vi "Limit Error.vi"(1 "Array":u8[](array[numeric])) -> (0 "LIMIT ERROR":bool)   [LabVIEW 2015]
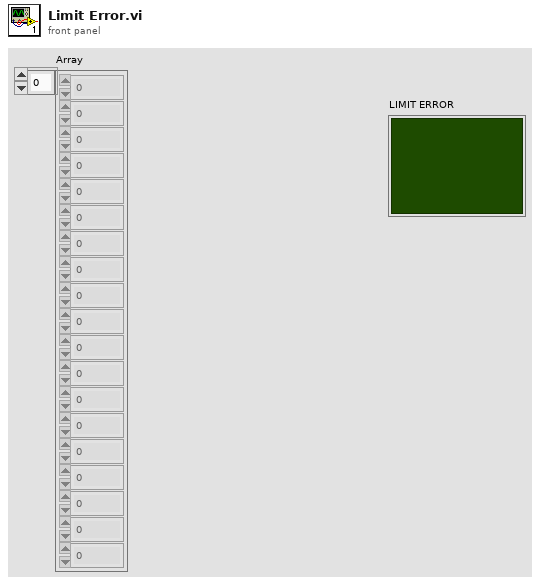
[diagram p1: front panel]
types:
  T1 = cluster{"Array[0]":u8, "Array[1]":u8, "Array[2]":u8, "Array[3]":u8, "Array[4]":u8, "Array[5]":u8, "Array[6]":u8, "Array[7]":u8, "Array[8]":u8, "Array[9]":u8, "Array[10]":u8, "Array[11]":u8, "Array[12]":u8, "Array[13]":u8, "Array[14]":u8, "Array[15]":u8, "Array[16]":u8, "Array[17]":u8, "Array[18]":u8}
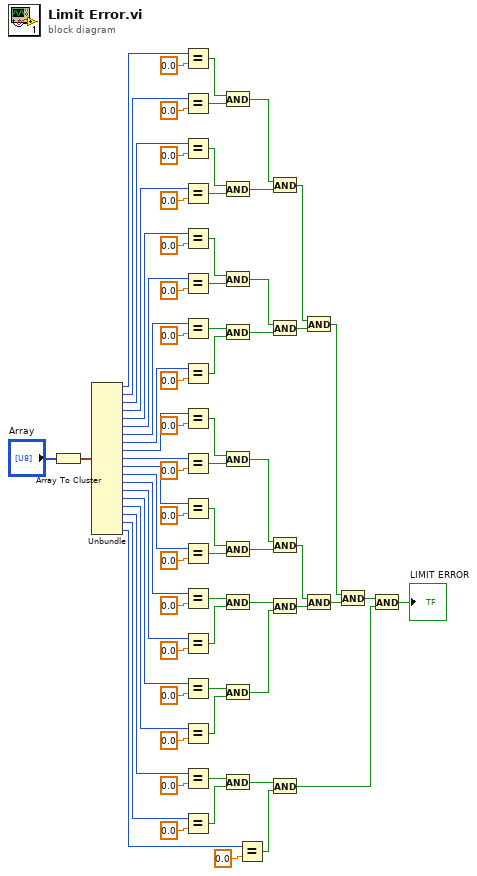
[diagram p0: block diagram]
diagram:
  n1 = Array To Cluster(array="Array") -> (cluster=w77:T1)
  n2 = Unbundle(w77) -> ("Array[0]"=w74:u8, "Array[1]"=w62:u8, "Array[2]"=w61:u8, "Array[3]"=w60:u8, "Array[4]"=w59:u8, "Array[5]"=w58:u8, "Array[6]"=w57:u8, "Array[7]"=w56:u8, "Array[8]"=w55:u8, "Array[9]"=w54:u8, "Array[10]"=w53:u8, "Array[11]"=w52:u8, "Array[12]"=w50:u8, "Array[13]"=w23:u8, "Array[14]"=w22:u8, "Array[15]"=w21:u8, "Array[16]"=w20:u8, "Array[17]"=w19:u8, "Array[18]"=w17:u8)
  n3 = Equal?(x=w74, y=0.0) -> (x = y?=w49:bool)
  n4 = Equal?(x=w62, y=0.0) -> (x = y?=w48:bool)
  n5 = Equal?(x=w61, y=0.0) -> (x = y?=w47:bool)
  n6 = Equal?(x=w60, y=0.0) -> (x = y?=w46:bool)
  n7 = Equal?(x=w59, y=0.0) -> (x = y?=w45:bool)
  n8 = Equal?(x=w58, y=0.0) -> (x = y?=w44:bool)
  n9 = Equal?(x=w57, y=0.0) -> (x = y?=w43:bool)
  n10 = Equal?(x=w56, y=0.0) -> (x = y?=w42:bool)
  n11 = Equal?(x=w55, y=0.0) -> (x = y?=w41:bool)
  n12 = Equal?(x=w54, y=0.0) -> (x = y?=w40:bool)
  n13 = Equal?(x=w53, y=0.0) -> (x = y?=w39:bool)
  n14 = Equal?(x=w52, y=0.0) -> (x = y?=w38:bool)
  n15 = Equal?(x=w50, y=0.0) -> (x = y?=w16:bool)
  n16 = Equal?(x=w23, y=0.0) -> (x = y?=w15:bool)
  n17 = Equal?(x=w22, y=0.0) -> (x = y?=w14:bool)
  n18 = Equal?(x=w21, y=0.0) -> (x = y?=w13:bool)
  n19 = Equal?(x=w20, y=0.0) -> (x = y?=w12:bool)
  n20 = Equal?(x=w19, y=0.0) -> (x = y?=w11:bool)
  n21 = And(x=w49, y=w48) -> (x .and. y?=w37:bool)
  n22 = And(x=w47, y=w46) -> (x .and. y?=w36:bool)
  n23 = And(x=w45, y=w44) -> (x .and. y?=w35:bool)
  n24 = And(x=w43, y=w42) -> (x .and. y?=w34:bool)
  n25 = And(x=w41, y=w40) -> (x .and. y?=w31:bool)
  n26 = And(x=w39, y=w38) -> (x .and. y?=w30:bool)
  n27 = And(x=w16, y=w15) -> (x .and. y?=w10:bool)
  n28 = And(x=w14, y=w13) -> (x .and. y?=w9:bool)
  n29 = And(x=w12, y=w11) -> (x .and. y?=w6:bool)
  n30 = Equal?(x=w17, y=0.0) -> (x = y?=w5:bool)
  n31 = And(x=w37, y=w36) -> (x .and. y?=w33:bool)
  n32 = And(x=w35, y=w34) -> (x .and. y?=w32:bool)
  n33 = And(x=w31, y=w30) -> (x .and. y?=w29:bool)
  n34 = And(x=w10, y=w9) -> (x .and. y?=w4:bool)
  n35 = And(x=w6, y=w5) -> (x .and. y?=w2:bool)
  n36 = And(x=w33, y=w32) -> (x .and. y?=w8:bool)
  n37 = And(x=w29, y=w4) -> (x .and. y?=w7:bool)
  n38 = And(x=w8, y=w7) -> (x .and. y?=w3:bool)
  n39 = And(x=w3, y=w2) -> (x .and. y?=→"LIMIT ERROR":bool)
